vi "Broadcast Data Source Info String.vi"(8 "error in (no error)":errorcluster, 10 "Data Source Info String":string, 11 "Application Manager in":refnum<class "Application Manager.lvclass">) -> (0 "error out":errorcluster, 3 "Application Manager out":refnum<class "Application Manager.lvclass">)   [LabVIEW 2020, in "Application Manager.lvlib" / "Application Manager.lvclass"]
uses:
  Application Manager.lvclass
  Application Manager.lvclass/Application Manager.ctl
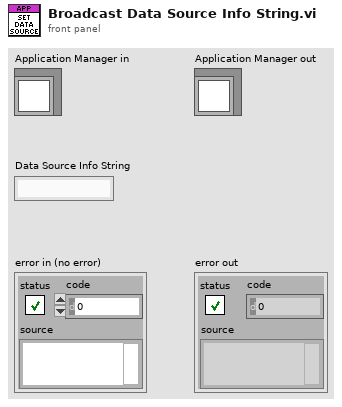
[diagram p1: front panel]
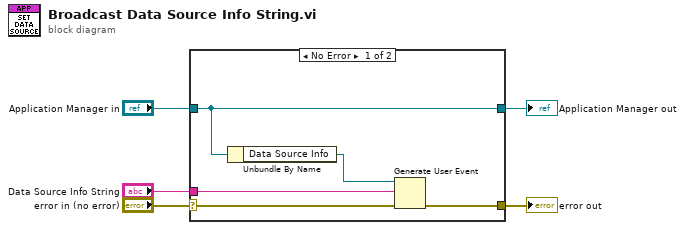
[diagram p0: block diagram]
diagram:
  n1 = case shown="No Error" "error in (no error)" {
    selector: "error in (no error)" -> [w10 w12]
    tunnel: [w8 w12] -> w4
    tunnel: [w7 w11] -> w2
    tunnel: "Application Manager in" -> [w7 w11]
    tunnel: "Data Source Info String" -> [w9 _]
    frame No Error {
      n2 = Unbundle By Name(w7) -> ("Data Source Info"=w6:refnum<user-event>)
      n3 = Generate User Event(user event=w6, event data cluster=w9, error in=w10) -> (error out=w8:errorcluster)  [unwired: 1 in, 1 out]
    }
    frame Error {
    }
  }
  "error out" <- w4
  "Application Manager out" <- w2
